vi "Begin Bin.vi"   [LabVIEW 2017, in "LabPack.lvlib" / "Reader.lvclass"]
uses:
  Reader.lvclass
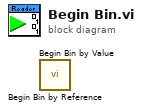
[diagram p0: block diagram]
diagram:
  n1 = call "Begin Bin by Reference.vi"() -> ()  [unwired: 9 in, 3 out]
  n2 = call "Begin Bin by Value.vi"() -> ()  [unwired: 9 in, 3 out]
